vi "File.Move All File and SubFolders from one Folder to Another Folder.vi"(8 "error in":errorcluster, 10 "Destination Folder":path, 11 "Source Folder":path) -> (0 "error out":errorcluster, 3 "Destination Out":path)   [LabVIEW 2024]
uses:
  Errors/Error.Error Code List.ctl
  <vilib>/KATE/Files/File Utils.lvlib
  Errors.lvlib
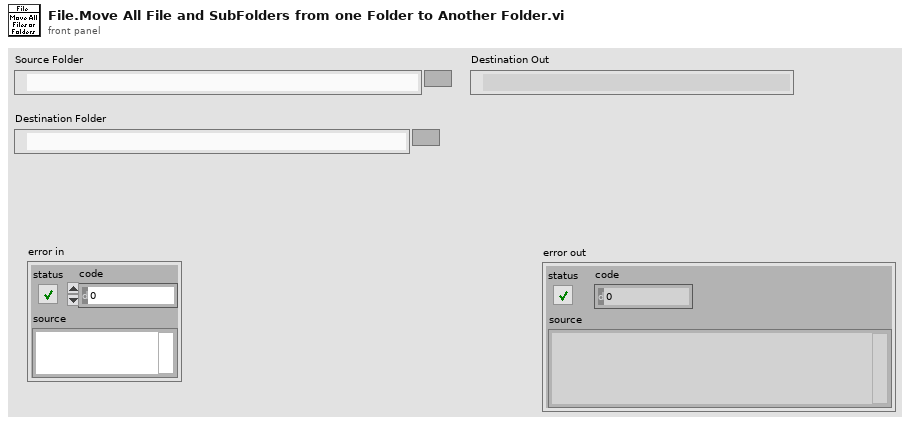
[diagram p1: front panel]
types:
  T1 = typedef "EQMF.lvlib/Errors.lvlib/Error.Error Code List.ctl" = i32
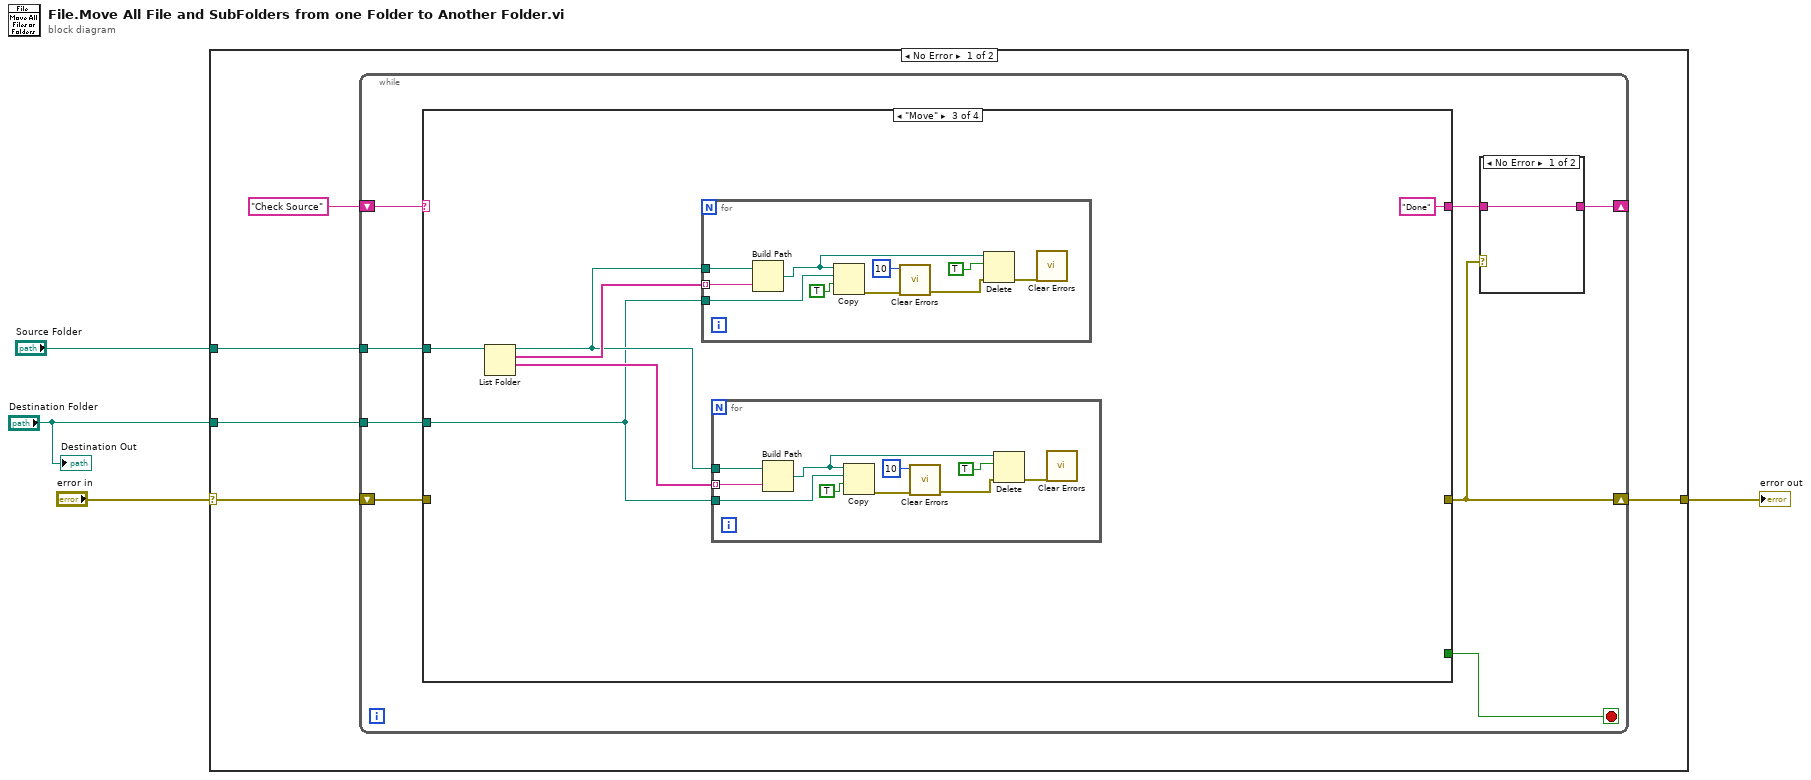
[diagram p0: block diagram]
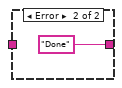
[diagram p2: hidden frame]
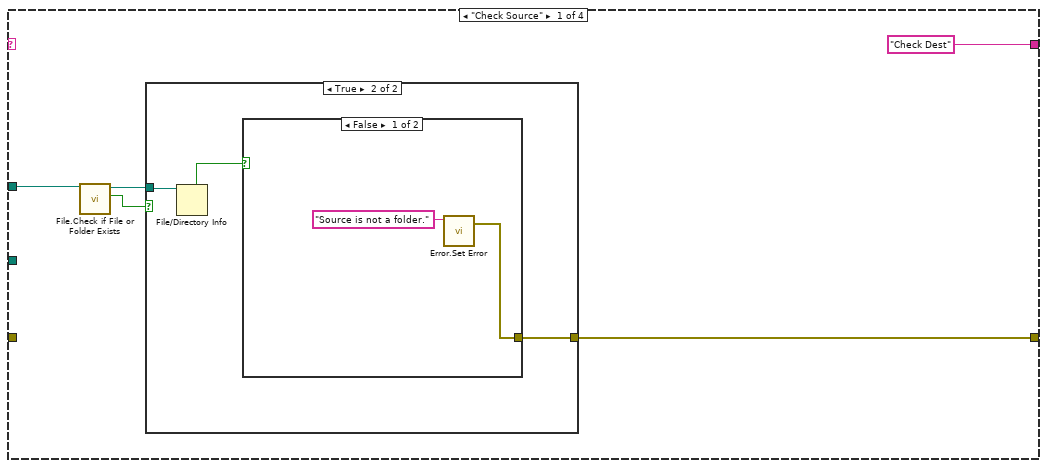
[diagram p3: hidden frame]
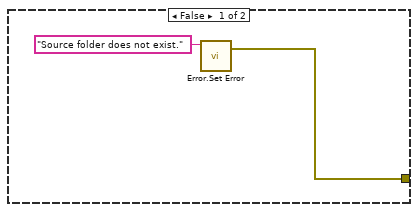
[diagram p4: hidden frame]
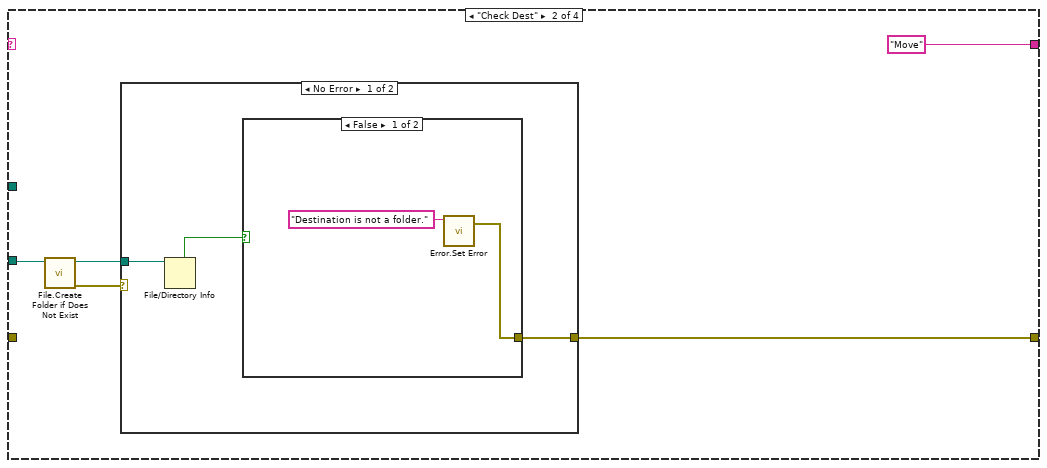
[diagram p6: hidden frame]
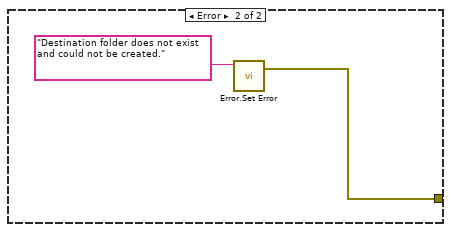
[diagram p8: hidden frame]
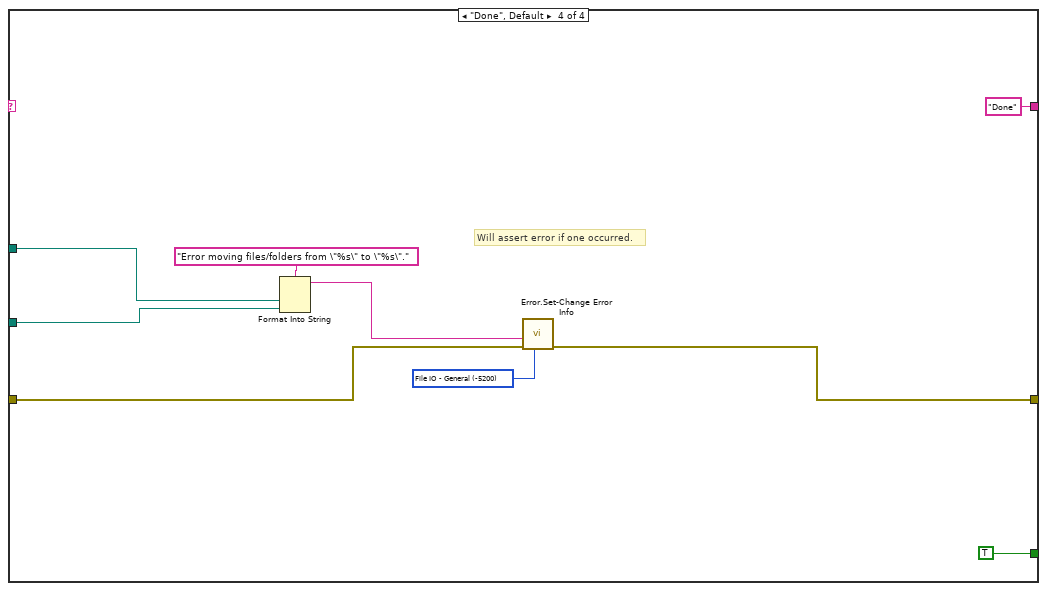
[diagram p9: hidden frame]
diagram:
  n1 = case shown="No Error" "error in" {
    selector: "error in" -> [w6 w79]
    tunnel: "Source Folder" -> [w9 _]
    tunnel: "Destination Folder" -> [w7 _]
    tunnel: [w5 w79] -> w2
    frame No Error {
      n2 = while {
        tunnel: w7 -> [w17]
        tunnel: w9 -> [w16]
        shift-right: [w12] -> _
        shift-left: "Check Source" -> [w14]
        shift-right: [w13] -> w5
        shift-left: w6 -> [w10]
        stop <- w15 stop-if-true
        n3 = case shown="\"Move\"" w14 {
          tunnel: w17 -> [_ w34 w44 w74]
          tunnel: w16 -> [w24 _ w48 w75]
          tunnel: [_ _ _ TRUE] -> w15
          tunnel: [w22 w36 _ w70] -> w13
          tunnel: ["Check Dest" "Move" "Done" "Done"] -> w11
          tunnel: w10 -> [_ _ _ w71]
          frame "Check Source" {
            n4 = call <vilib>:"File.Check if File or Folder Exists.vi"("Path"=w24) -> ("Exists"=w23:bool, "Dup Path"=w20:path)  [unwired: 6 in, 3 out]
            n5 = case shown="True" w23 {
              tunnel: [w25 w27] -> w22
              tunnel: w20 -> [_ w29]
              frame False {
                n6 = call "Error.Set Error.vi"("Desc"="Source folder does not exist.") -> ("error out"=w25:errorcluster)  [unwired: 6 in]
              }
              frame True {
                n7 = File/Directory Info(path=w29) -> (directory=w28:bool)  [unwired: 1 in, 6 out]
                n8 = case shown="False" w28 {
                  tunnel: [w30 _] -> w27
                  frame False {
                    n9 = call "Error.Set Error.vi"("Desc"="Source is not a folder.") -> ("error out"=w30:errorcluster)  [unwired: 6 in]
                  }
                  frame True {
                  }
                }
              }
            }
          }
          frame "Check Dest" {
            n10 = call <vilib>:"File.Create Folder if Does Not Exist.vi"("Path"=w34) -> ("error out"=w32:errorcluster, "Dup Path"=w33:path)  [unwired: 8 in, 1 out]
            n11 = case shown="No Error" w32 {
              tunnel: [w37 w42] -> w36
              tunnel: w33 -> [w39 _]
              frame No Error {
                n12 = File/Directory Info(path=w39) -> (directory=w38:bool)  [unwired: 1 in, 6 out]
                n13 = case shown="False" w38 {
                  tunnel: [w40 _] -> w37
                  frame False {
                    n14 = call "Error.Set Error.vi"("Desc"="Destination is not a folder.") -> ("error out"=w40:errorcluster)  [unwired: 6 in]
                  }
                  frame True {
                  }
                }
              }
              frame Error {
                n15 = call "Error.Set Error.vi"("Desc"="Destination folder does not exist and could not be created.") -> ("error out"=w42:errorcluster)  [unwired: 6 in]
              }
            }
          }
          frame "Move" {
            n16 = List Folder(path=w48) -> (path out=w46:path, filenames=w47:string[], folder names=w45:string[])  [unwired: 3 in, 1 out]
            n17 = for {
              tunnel: w46 -> [w64]
              tunnel: w47 -> [w63] mode=indexing
              tunnel: w44 -> [w61]
              n18 = Build Path(base path=w64, name or relative path=w63) -> (appended path=w62:path)
              n19 = Copy(9:TRUE ("overwrite (F)"), 10:w61, 11:w62) -> (0:w69:errorcluster)  [unwired: 2 in, 2 out]
              n20 = call <vilib>:"Clear Errors.vi"("error in (no error)"=w69, "specific error code to clear (0: all)"=10) -> ("error out"=w68:errorcluster)  [unwired: 4 in, 1 out]
              n21 = Delete(path (use dialog)=w62, entire hierarchy (F)=TRUE, error in=w68) -> (error out=w60:errorcluster)  [unwired: 2 in, 2 out]
              n22 = call <vilib>:"Clear Errors.vi"("error in (no error)"=w60) -> ()  [unwired: 5 in, 2 out]
            }
            n23 = for {
              tunnel: w46 -> [w54]
              tunnel: w45 -> [w53] mode=indexing
              tunnel: w44 -> [w51]
              n24 = Build Path(base path=w54, name or relative path=w53) -> (appended path=w52:path)
              n25 = Copy(9:TRUE ("overwrite (F)"), 10:w51, 11:w52) -> (0:w59:errorcluster)  [unwired: 2 in, 2 out]
              n26 = call <vilib>:"Clear Errors.vi"("error in (no error)"=w59, "specific error code to clear (0: all)"=10) -> ("error out"=w58:errorcluster)  [unwired: 4 in, 1 out]
              n27 = Delete(path (use dialog)=w52, entire hierarchy (F)=TRUE, error in=w58) -> (error out=w50:errorcluster)  [unwired: 2 in, 2 out]
              n28 = call <vilib>:"Clear Errors.vi"("error in (no error)"=w50) -> ()  [unwired: 5 in, 2 out]
            }
          }
          frame "Done", Default {
            w76 = T1 -5200 items=["No Error"=0, "Abort"=-2, "Misc"=-5000, "Fixture Error"=-5100, "File IO - General"=-5200, "FIle IO - Config Error"=-5201, "Instrument - General"=-5300, "Instrument - Serial Com"=-5301, "Instrument - Camera"=-5302, "Instrument - PS"=-5303, "Instrument - Oscilloscope"=-5304, "Instrument - Function Gen"=-5305, "Instrument - Load"=-5306, "Instrument - Meter"=-5307, "Instrument - Power Control"=-5308, "Instrument - Motion"=-5309, "Instrument - RF"=-5310, "System Exe"=-5400, "Image Processing"=-5500, "Communication"=-5600, "Script - Syntax Error"=-6000, "Script - Invalid Name or Param"=-6100, "Script - Timeout"=-6200, "Invalid Data"=-6300, "FW Update Error"=-6500] ("Std Code")
            # "Will assert error if one occurred."
            n29 = Format Into String(format string="Error moving files/folders from \"%s\" to \"%s\".", w75, w74) -> (resulting string=w73:string)  [unwired: 2 in, 1 out]
            n30 = call "Error.Set-Change Error Info.vi"("Std Code"=w76, "error in"=w71, "Description"=w73) -> ("error out"=w70:errorcluster)  [unwired: 8 in]
          }
        }
        n31 = case shown="No Error" w13 {
          tunnel: [w18 "Done"] -> w12
          tunnel: w11 -> [w18 _]
          frame No Error {
          }
          frame Error {
          }
        }
      }
    }
    frame Error {
    }
  }
  "error out" <- w2
  "Destination Out" <- "Destination Folder"
